vi "Pattern recognition.vi"(9 "Template Path":path, 10 "Minimum match points":i32, 11 "Image 2":T2(plugin-control)) -> (2 "Image":T2(plugin-control), 3 "Matches (pixel)":T1(array[cluster]))   [LabVIEW 2015]
uses:
  <vilib>/vision/NI_Vision_Development_Module.lvlib
panel:
  out "Number of Matches Found":i32
  in  "Advanced Options":cluster{"Item":u16, "Value":dbl}[](array[cluster])=[{"Item"=1, "Value"=1.0}, {"Item"=103, "Value"=1.0}] {"Item" items=["LD Sampling - Minimum Constrast"=0, "LD Sampling - Enable Subpixel Accuracy"=1, "LD Sampling - Search Strategy"=2, "LD Sampling - Subpixel Iterations"=3, "LD Sampling - Subpixel Tolerance"=4, "LD Sampling - Initial Match List Length"=5, "LD Sampling - Match List Reduction Factor"=6, "LD Sampling - Initial Step Size"=7, "LD Sampling - Intermediate Angular Accuracy"=8, "-"=9, "Pyramid - Max Pyramid Level"=100, "Pyramid - Minimum Contrast"=102, "Pyramid - Enable Subpixel Accuracy"=103, "Pyramid - Subpixel Iterations"=104, "Pyramid - Subpixel Tolerance"=105, "Pyramid - Initial Match List Length"=106, "Pyramid - Match List Reduction Factor"=107, "Pyramid - Intermediate Angular Accuracy"=108, "Pyramid - Process Border Matches"=109, "Pyramid - Min Match Separation Distance"=111, "Pyramid - Min Match Separation Angle"=112, "Pyramid - Max Match Overlap"=113, "Pyramid - Max Cache in MB"=114, "Pyramid - Clear Cache"=115]}
  in  "Match Parameters":T3={"Number of Matches Requested"=1, "Minimum Match Score"=750.0, "Angle Ranges"=[]} {"Angle Ranges"."End Angle" min=-360 max=360; "Angle Ranges"."Start Angle" min=-360 max=360; "Minimum Match Score" min=0 max=1000; "Number of Matches Requested" min=1 max=9999}
  in  "Algorithm":i32(ring)=2 items=["All", "Low Discrepancy Sampling", "Grayscale Value Pyramid", "Gradients Pyramid"]
  out "Elapsed Time (ms)":dbl format="%.2f"
  out "Matches":T1(array[cluster]) {"Bounding Box"."y" format="%.2g"; "Bounding Box"."x" format="%.2g"; "Score" format="%.2f"; "Scale" format="%.2g"; "Angle" format="%.2g"; "Position"."y" format="%.2g"; "Position"."x" format="%.2g"}
  out "Template Report":T4={"Template Contrast"=0, "Grayvalue Max Pyramid Level"=-1, "Grayvalue Optimal Pyramid Level"=-1, "Gradient Max Pyramid Level"=-1, "Gradient Optimal Pyramid Level"=-1}
  out "Template":T2(plugin-control)
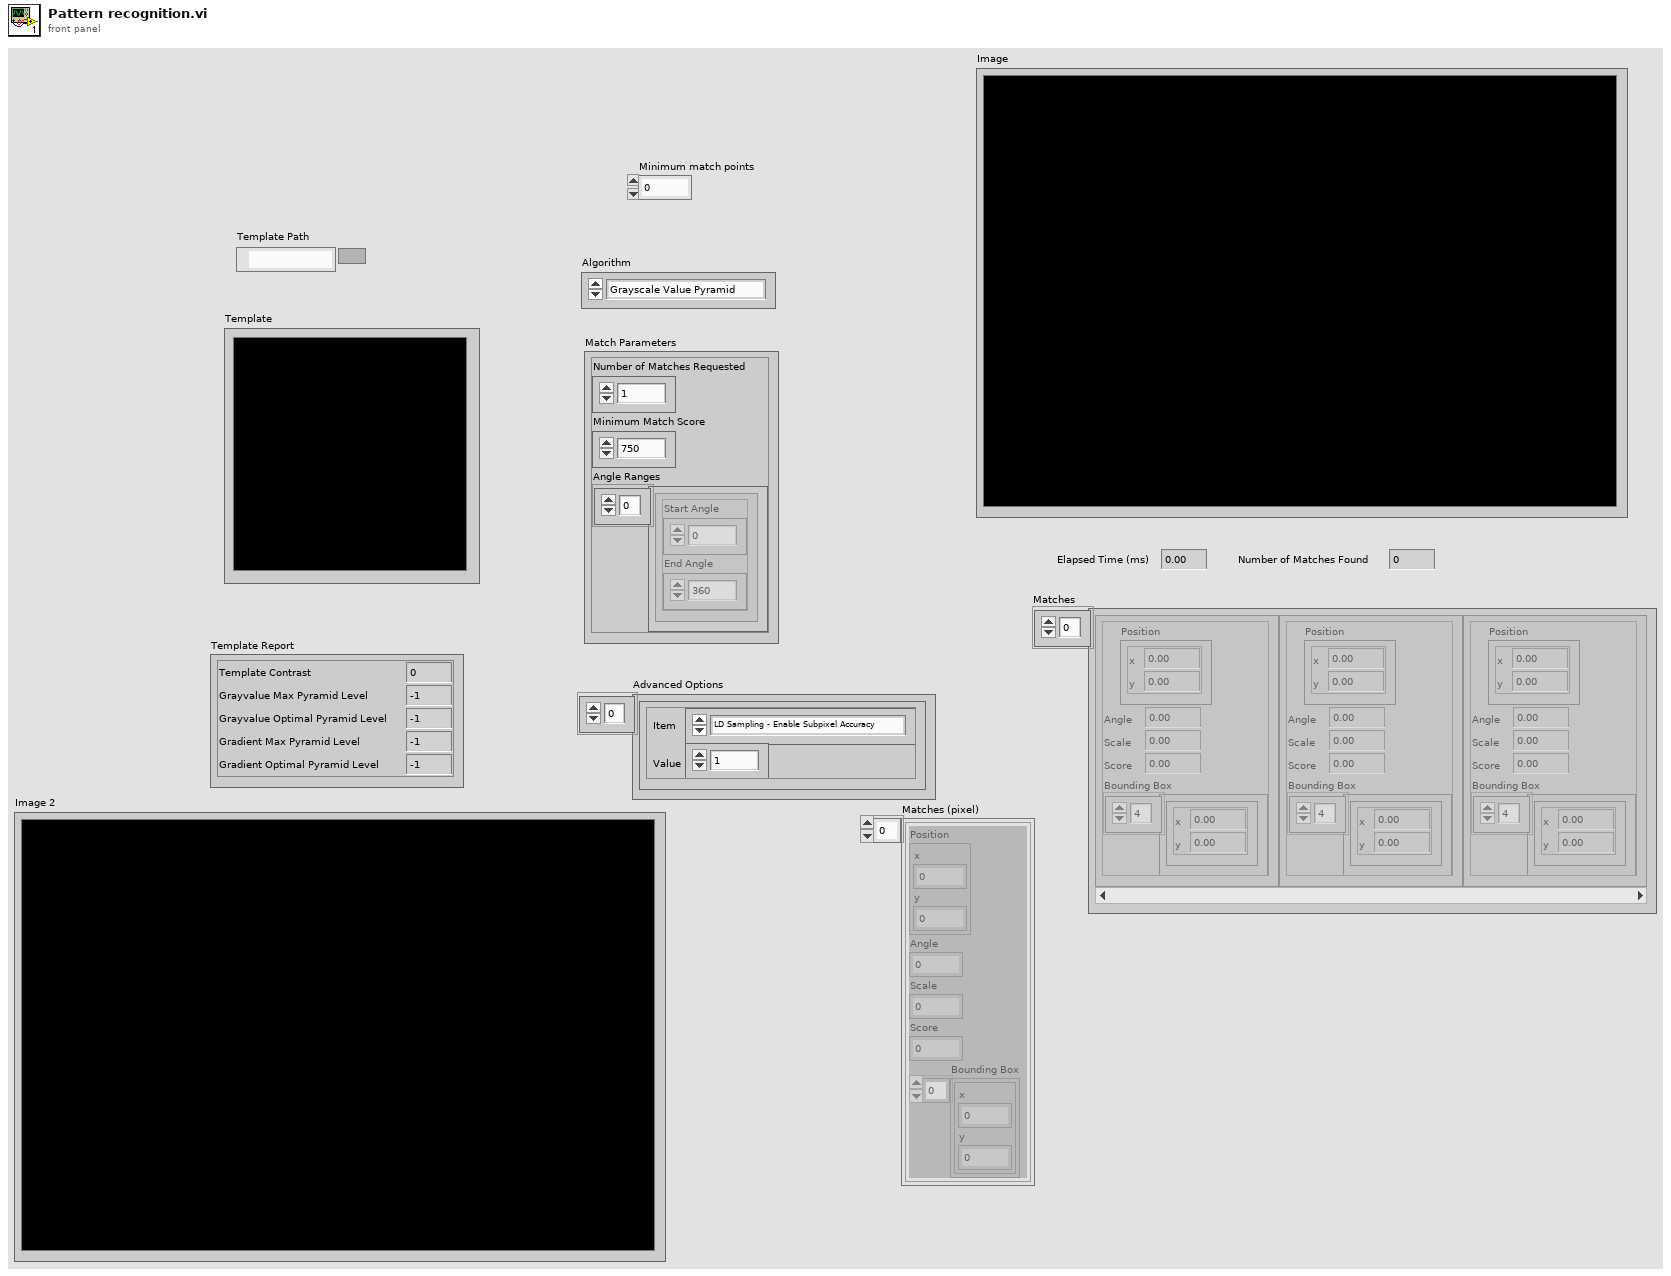
[diagram p1: front panel]
types:
  T1 = cluster{"Position":cluster{"x":sgl, "y":sgl}, "Angle":sgl, "Scale":sgl, "Score":sgl, "Bounding Box":cluster{"x":sgl, "y":sgl}[]}[]
  T2 = typedef "IMAQ Image.ctl" = refnum<image>
  T3 = cluster{"Number of Matches Requested":i32, "Minimum Match Score":sgl, "Angle Ranges":cluster{"Start Angle":sgl, "End Angle":sgl}[]}
  T4 = cluster{"Template Contrast":i32, "Grayvalue Max Pyramid Level":i32, "Grayvalue Optimal Pyramid Level":i32, "Gradient Max Pyramid Level":i32, "Gradient Optimal Pyramid Level":i32}
  T5 = cluster{"Number of Matches Requested":i32, "Minimum match points":i32, "Angle Ranges":cluster{"Start Angle":sgl, "End Angle":sgl}[]}
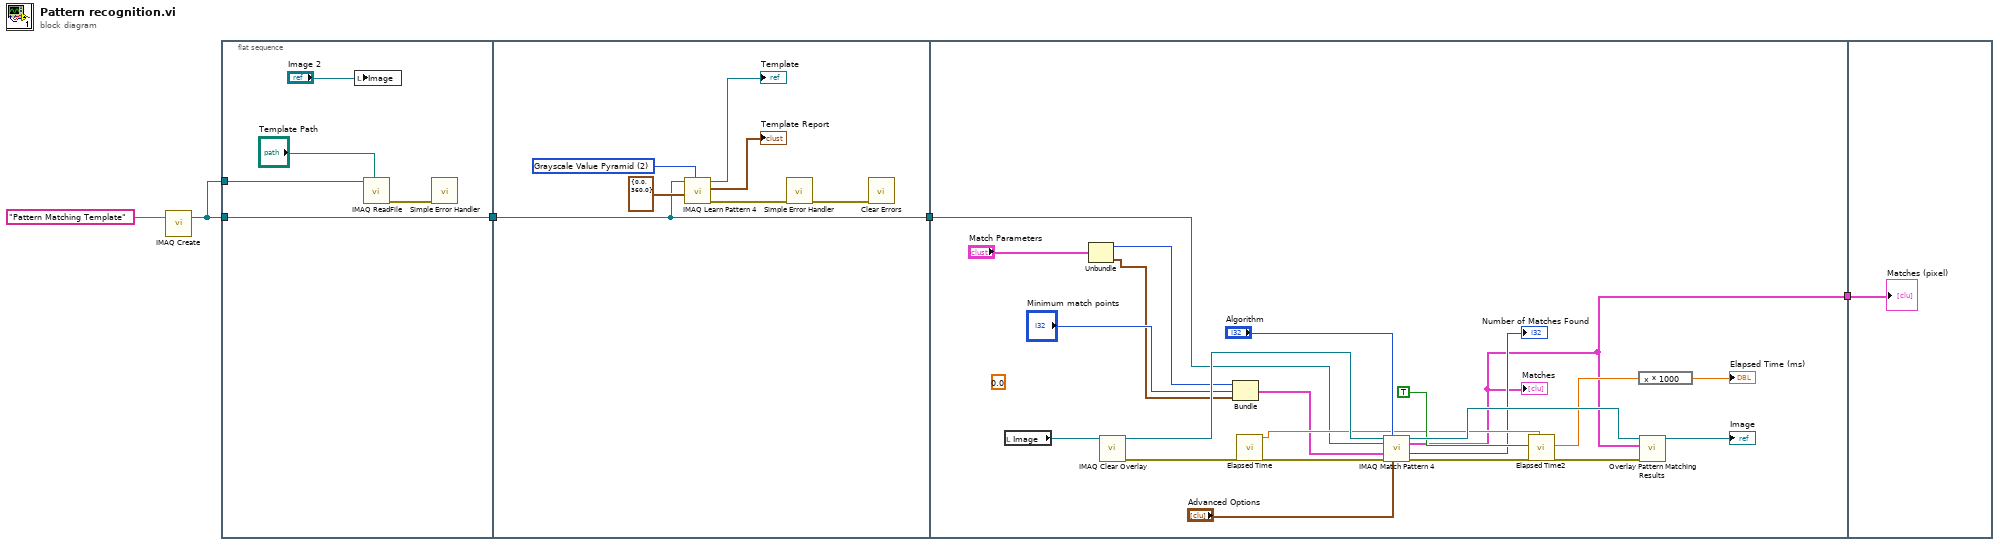
[diagram p0: block diagram]
diagram:
  n1 = call "IMAQ Create"("Image Name"="Pattern Matching Template") -> ("New Image"=w4:T2)  [unwired: 4 in, 1 out]
  n2 = flat-sequence {
    tunnel: w4 -> [w8]
    tunnel: w4 -> [w7]
    tunnel: [w7] -> w3
    tunnel: w3 -> [w11]
    tunnel: [w11] -> w2
    tunnel: w2 -> [w25]
    tunnel: [w19] -> w1
    tunnel: w1 -> [w40]
    frame #0 {
      n3 = local write "Image"("Image 2") -> ()
      n4 = call "IMAQ ReadFile"("File Path"="Template Path", "Image"=w8) -> ("error out"=w10:errorcluster)  [unwired: 5 in, 4 out]
      n5 = call <vilib>:"Simple Error Handler.vi"("error in (no error)"=w10) -> ()  [unwired: 4 in, 5 out]
    }
    frame #1 {
      w17 = 2 items=["All", "Low Discrepancy Sampling", "Grayscale Value Pyramid", "Gradients Pyramid"] ("Algorithm")
      n6 = call "IMAQ Learn Pattern 4"("Algorithm"=w17, "Angle Range"=cluster{"Start Angle":sgl, "End Angle":sgl} {"Start Angle"=0.0, "End Angle"=360.0}, "Image"=w11) -> ("error out"=w14:errorcluster, "Template Report"=→"Template Report":T4, "Template Image Out"=→"Template":T2)  [unwired: 6 in]
      n7 = call <vilib>:"Simple Error Handler.vi"("error in (no error)"=w14) -> ("error out"=w13:errorcluster)  [unwired: 4 in, 4 out]
      n8 = call <vilib>:"Clear Errors.vi"("error in (no error)"=w13) -> ()  [unwired: 5 in, 2 out]
    }
    frame #2 {
      (unwired) sgl 0.0
      n9 = local read "Image"() -> (w20:T2)
      n10 = Unbundle("Match Parameters") -> ("Number of Matches Requested"=w23:i32, "Angle Ranges"=w18:cluster{"Start Angle":sgl, "End Angle":sgl}[])  [unwired: 1 out]
      n11 = call "IMAQ Clear Overlay"("Image"=w20) -> ("error out"=w33:errorcluster, "Image Out"=w36:T2)  [unwired: 9 in]
      n12 = Bundle("Number of Matches Requested"=w23, "Minimum match points"="Minimum match points", "Angle Ranges"=w18) -> (w21:T5)  [unwired: 1 in]
      n13 = call "Elapsed Time"("error in (no error)"=w33) -> ("Present (s)"=w28:dbl, "error out"=w32:errorcluster)  [unwired: 11 in, 6 out]
      n14 = call "IMAQ Match Pattern 4"("Image"=w36, "Algorithm"="Algorithm", "Template Image"=w25, "Parameters"=w21, "error in (no error)"=w32, "Advanced Options"="Advanced Options") -> ("Image (duplicate)"=w38:T2, "Matches (pixel)"=w19:T1, "Number of Matches"=→"Number of Matches Found":i32, "error out"=w31:errorcluster)  [unwired: 5 in, 1 out]
      "Matches" <- w19
      n15 = call "Elapsed Time2"("Reset"=TRUE, "error in (no error)"=w31, "Set Start Time (s)"=w28) -> ("Elapsed Time (s)"=w35:dbl, "error out"=w29:errorcluster)  [unwired: 9 in, 6 out]
      n16 = expression code="x * 1000"(w35) -> (→"Elapsed Time (ms)":dbl)
      n17 = call "Overlay Pattern Matching Results.vi"("error in"=w29, "Matches"=w19, "Image"=w38) -> ("Image Out"=→"Image":T2)  [unwired: 7 in, 1 out]
    }
    frame #3 {
      "Matches (pixel)" <- w40
    }
  }
